vi "looptunnel.vi"() -> ()   [LabVIEW 2021]
panel:
  in  "Numeric 6":dbl
  in  "Numeric 5":dbl
  out "Numeric 4":i32
  out "x+y 2":dbl
  in  "Stop 2":bool
  in  "Stop":bool
  out "x+y":dbl
  in  "Numeric 3":dbl
  in  "Numeric 2":dbl
  out "Numeric":i32
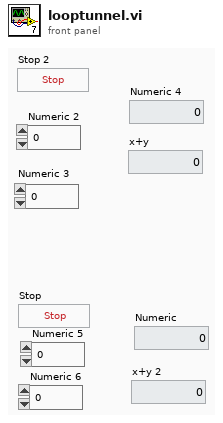
[diagram p1: front panel]
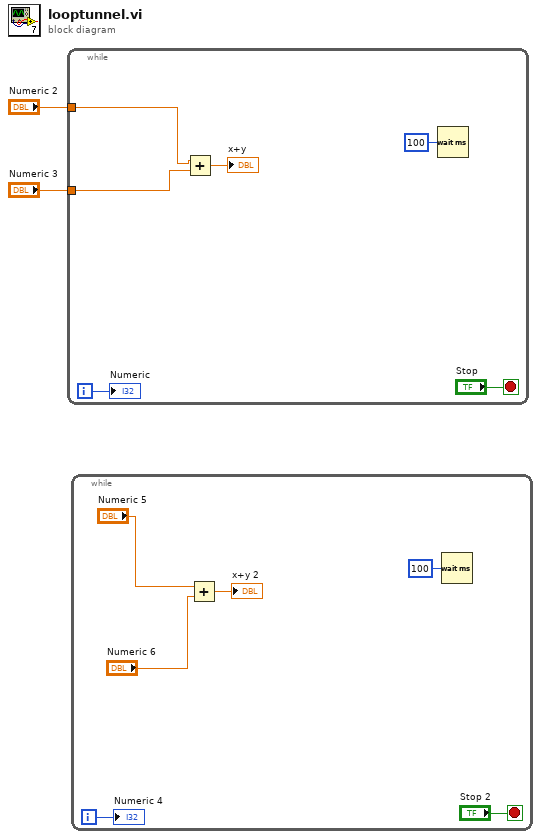
[diagram p0: block diagram]
diagram:
  n1 = while {
    tunnel: "Numeric 2" -> [w6]
    tunnel: "Numeric 3" -> [w5]
    i -> [w7]
    stop <- "Stop" stop-if-true
    n2 = Add(x=w6, y=w5) -> (x+y=→"x+y":dbl)
    n3 = Wait (ms)(milliseconds to wait=u32 100) -> ()  [unwired: 1 out]
    "Numeric" <- w7
  }
  n4 = while {
    i -> [w13]
    stop <- "Stop 2" stop-if-true
    n5 = Add(x="Numeric 5", y="Numeric 6") -> (x+y=→"x+y 2":dbl)
    n6 = Wait (ms)(milliseconds to wait=u32 100) -> ()  [unwired: 1 out]
    "Numeric 4" <- w13
  }
